vi "dust_event_query.vi"(6 "No. of Events":u64=10, 8 "error in (no error)":errorcluster, 9 "Limited?":bool, 10 "Small?":bool, 11 "Constraints":T4 {"Estimate Quality" scale=0.0..5.0; "Lower Mass Limit (kg)" min=-1.0 max=1.0 step=1e-20; "Upper Mass Limit (kg)" min=-1.0 max=1.0 step=1e-20; "Lower Velocity Limit (km/s)" min=-1.0 max=299792000.0; "Upper Velocity Limit (km/s)" min=-1.0 max=299792000.0}) -> (0 "error out":errorcluster, 1 "Experiment Settings ID Array":i32[](array[numeric]), 2 "Dust Event ID Array":i64[](array[numeric]), 3 "Dust Array":T1[](array[typedef]) {"File Location" items=["Unknown"=-1, "Processing"=0, "Storage"=1]; "Estimate Source" items=["Any Source."=-2, "No Shot"=-1, "Basic Labview Estimate"=0, "IDL Estimate From Andrew"=1, "IDL Estimate From Tobin"=2, "Old Metadata"=3]}, 5 "File Location Array":i8[](array[numeric]))   [LabVIEW 2013]
doc: "Given a set of constraints, this program will return a lot of data about each event that matches the constraints."
uses:
  User Interface/Controls/Constraints.ctl
  User Interface/Controls/Query_Dust_Event.ctl
  User Interface/Controls/Estimate_source.ctl
  User Interface/Controls/File_location.ctl
  <userlib>/_OpenG.lib/array/array.llb/Reverse 2D Array (Variant)__ogtk.vi
  <vilib>/addons/database/_DB Variant To Data/Database Variant To Data.xnode
panel:
  out "SQL Query Syntax":string
  # "Dust Event"
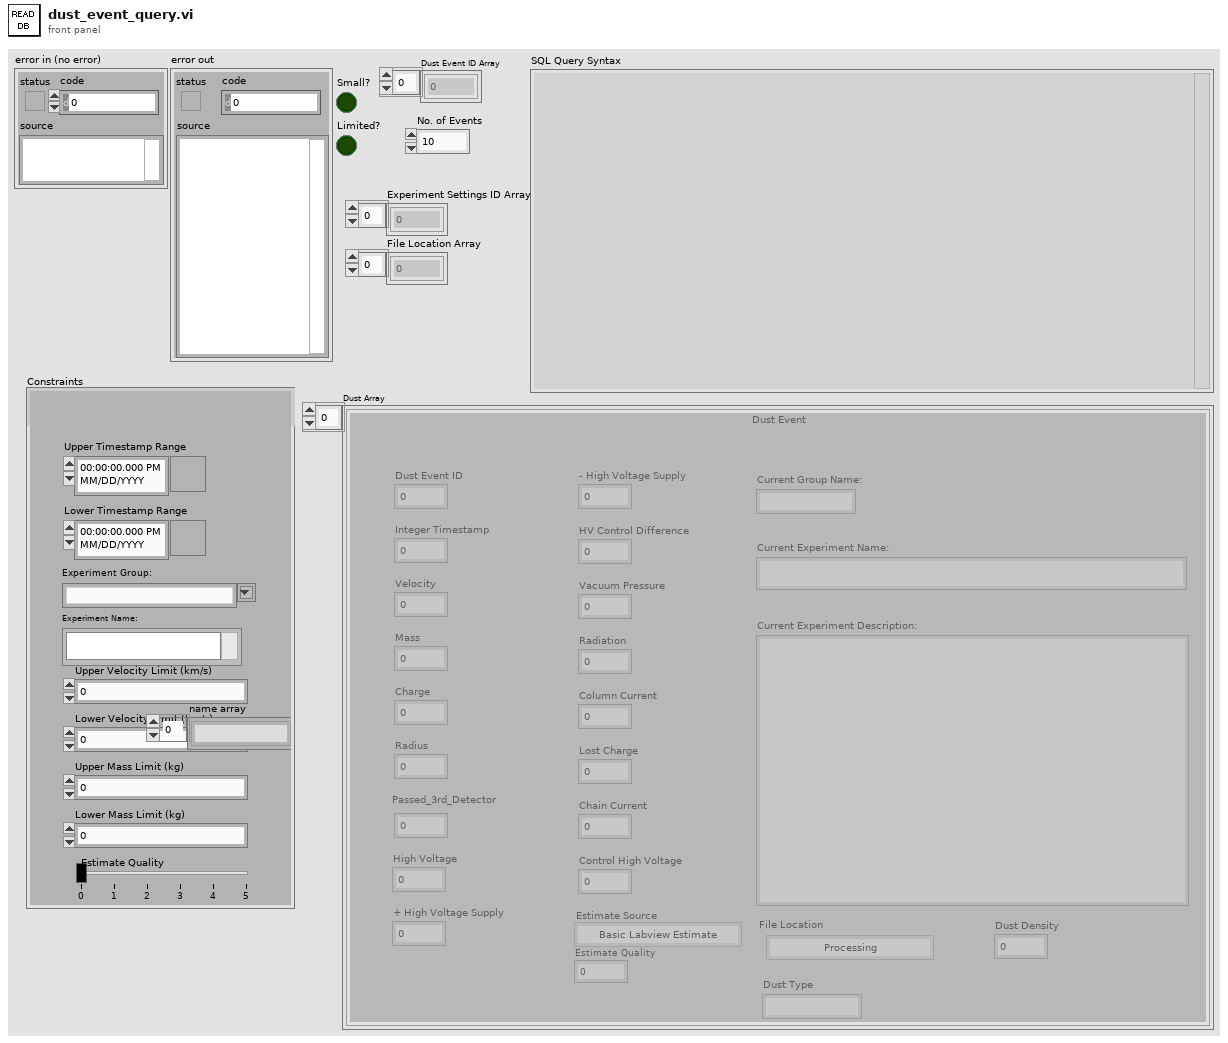
[diagram p1: front panel]
types:
  T1 = typedef "Query_Dust_Event.ctl" = cluster{"Dust Event ID":i64, "Integer Timestamp":i64, "Velocity":dbl, "Mass":dbl, "Charge":sgl, "Radius":sgl, "Passed_3rd_Detector":i8, "High Voltage":sgl, "+ High Voltage Supply":sgl, "- High Voltage Supply":sgl, "HV Control Difference":sgl, "Vacuum Pressure":sgl, "Radiation":sgl, "Column Current":sgl, "Lost Charge":sgl, "Chain Current":sgl, "Control High Voltage":sgl, "Current Group Name:":string, "Current Experiment Name:":string, "Current Experiment Description:":string, "Estimate Source":T2, "Estimate Quality":i8, "File Location":T3, "Dust Type":string, "Dust Density":sgl}
  T2 = typedef "Estimate_source.ctl" = i8
  T3 = typedef "File_location.ctl" = i8
  T4 = typedef "Constraints.ctl" = cluster{"Upper Timestamp Range":timestamp, "Lower Timestamp Range":timestamp, "Experiment Group:":string, "Experiment Name:":i32[], "Upper Velocity Limit (km/s)":dbl, "Lower Velocity Limit (km/s)":dbl, "Upper Mass Limit (kg)":dbl, "Lower Mass Limit (kg)":dbl, "name array":string[], "Estimate Quality":cluster{dbl, dbl}}
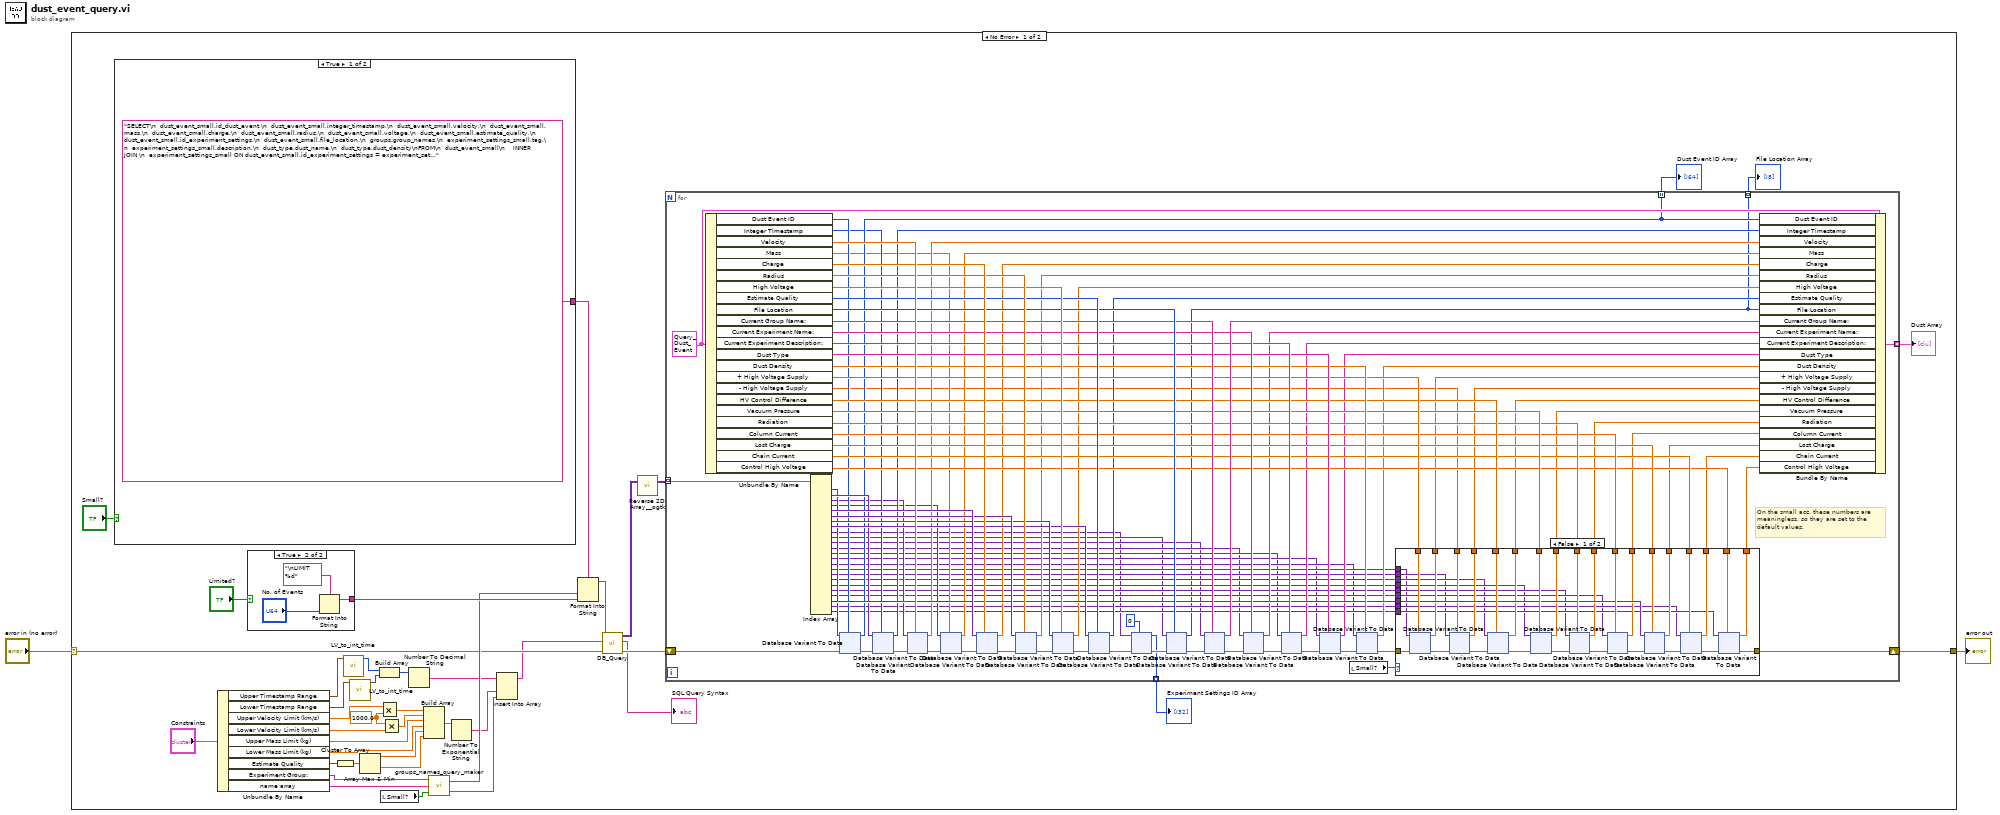
[diagram p0: block diagram]
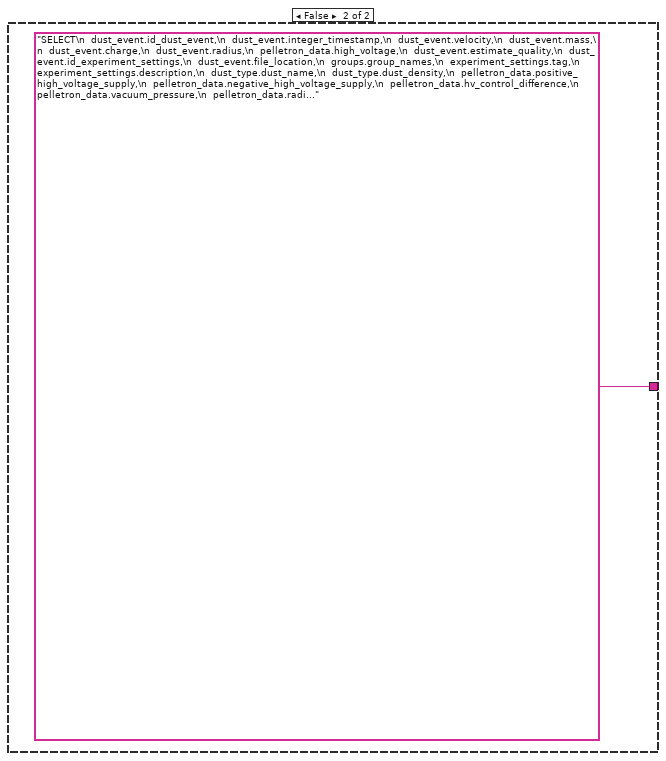
[diagram p3: hidden frame]
diagram:
  n1 = case shown="No Error" "error in (no error)" {
    selector: "error in (no error)" -> [w17 w957]
    tunnel: [w38 w957] -> w1
    frame No Error {
      w23 = 1000.0 ("y")
      n2 = case shown="True" "Small?" {
        tunnel: ["SELECT\n  dust_event_small.id_dust_event,\n  dust_event_small.integer_timestamp,\n  dust_event_small.velocity,\n  dust_event_small.mass,\n  dust_event_small.charge,\n  dust_event_small.radius,\n  dust_event_small.voltage,\n  dust_event_small.estimate_quality,\n  dust_event_small.id_experiment_settings,\n  dust_event_small.file_location,\n  groups.group_names,\n  experiment_settings_small.tag,\n  experiment_settings_small.description,\n  dust_type.dust_name,\n  dust_type.dust_density\nFROM\n  dust_event_small\n    INNER JOIN \n  experiment_settings_small ON dust_event_small.id_experiment_settings = experiment_settings_small.id_experiment_settings\n    INNER JOIN  \n  groups ON experiment_settings_small.id_groups=groups.id_groups\n    INNER JOIN\n  dust_info_small ON dust_event_small.id_dust_info = dust_info_small.id_dust_info\n  \t\tINNER JOIN\n  dust_type ON dust_info_small.dust_type = dust_type.id_dust_type\nWHERE\n  dust_event_small.integer_timestamp <= ? AND dust_event_small.integer_timestamp >= ?\n    AND\n  dust_event_small.velocity <= ? AND dust_event_small.velocity >= ?\n    AND\n  dust_event_small.mass <= ? AND dust_event_small.mass >= ?\n    AND\n  dust_event_small.estimate_quality <= ? AND dust_event_small.estimate_quality >= ?%s\nORDER BY\n  dust_event_small.id_dust_event DESC%s; " ("string") "SELECT\n  dust_event.id_dust_event,\n  dust_event.integer_timestamp,\n  dust_event.velocity,\n  dust_event.mass,\n  dust_event.charge,\n  dust_event.radius,\n  pelletron_data.high_voltage,\n  dust_event.estimate_quality,\n  dust_event.id_experiment_settings,\n  dust_event.file_location,\n  groups.group_names,\n  experiment_settings.tag,\n  experiment_settings.description,\n  dust_type.dust_name,\n  dust_type.dust_density,\n  pelletron_data.positive_high_voltage_supply,\n  pelletron_data.negative_high_voltage_supply,\n  pelletron_data.hv_control_difference,\n  pelletron_data.vacuum_pressure,\n  pelletron_data.radiation,\n  pelletron_data.column_current,\n  pelletron_data.lost_charge,\n  pelletron_data.chain_current,\n  pelletron_data.control_high_voltage\nFROM\n  dust_event\n    INNER JOIN \n  experiment_settings ON dust_event.id_experiment_settings = experiment_settings.id_experiment_settings\n    INNER JOIN  \n  groups ON experiment_settings.id_groups=groups.id_groups\n    INNER JOIN\n  pelletron_data ON pelletron_data.id_pelletron_data = dust_event.id_pelletron_data\n    INNER JOIN\n  dust_info ON dust_event.id_dust_info = dust_info.id_dust_info\n\t\t  INNER JOIN\n\t dust_type ON dust_info.dust_type = dust_type.id_dust_type\nWHERE\n  dust_event.integer_timestamp <= ?  AND dust_event.integer_timestamp >= ?\n    AND\n  dust_event.velocity <= ?  AND dust_event.velocity >= ?\n    AND\n  dust_event.mass <= ?  AND dust_event.mass >= ?\n    AND\n  dust_event.estimate_quality <= ? AND dust_event.estimate_quality >= ?%s\nORDER BY\n  dust_event.id_dust_event DESC%s; " ("string")] -> w29
        frame True {
        }
        frame False {
        }
      }
      n3 = Unbundle By Name("Constraints") -> ("Upper Timestamp Range"=w37:timestamp, "Lower Timestamp Range"=w36:timestamp, "Upper Velocity Limit (km/s)"=w35:dbl, "Lower Velocity Limit (km/s)"=w22:dbl, "Upper Mass Limit (kg)"=w11:dbl, "Lower Mass Limit (kg)"=w12:dbl, "Estimate Quality"=w24:cluster{dbl, dbl}, "Experiment Group:"=w26:string, "name array"=w25:string[])
      n4 = case shown="True" "Limited?" {
        tunnel: [_ w44] -> w28
        frame False {
        }
        frame True {
          n5 = Format Into String(format string="\nLIMIT %d", "No. of Events") -> (resulting string=w44:string)  [unwired: 2 in, 1 out]
        }
      }
      n6 = Cluster To Array(cluster=w24) -> (array=w40:dbl[])
      n7 = call "LV_to_int_time.vi"("Time Stamp"=w37) -> ("Integer Time"=w10:i64)  [unwired: 8 in, 1 out]
      n8 = call "LV_to_int_time.vi"("Time Stamp"=w36) -> ("Integer Time"=w9:i64)  [unwired: 8 in, 1 out]
      n9 = Array Max & Min(array=w40) -> (max value=w13:dbl, min value=w14:dbl)  [unwired: 2 out]
      n10 = Build Array(w10, w9) -> (w7:i64[])
      n11 = Multiply(x=w35, y=w23) -> (x*y=w16:dbl)
      n12 = local read "Small?"() -> (w18:bool)
      n13 = Multiply(x=w23, y=w22) -> (x*y=w15:dbl)
      n14 = Number To Decimal String(number=w7) -> (decimal integer string=w6:string[])  [unwired: 1 in]
      n15 = Build Array(w16, w15, w11, w12, w13, w14) -> (w8:dbl[])
      n16 = call "groups_names_query_maker.vi"("Small?"=w18, "Name Array"=w25, "Group  Name"=w26) -> ("Parameters"=w5:string[], "Group and Names Query"=w27:string)
      n17 = Number To Exponential String(number=w8) -> (E-format string=w4:string[])  [unwired: 3 in]
      n18 = Insert Into Array(array=w6, new element #1=w4, new element #2=w5) -> (w3:string[])  [unwired: 1 in]
      n19 = Format Into String(format string=w29, w27, w28) -> (resulting string=w21:string)  [unwired: 2 in, 1 out]
      n20 = call "DB_Query.vi"("error in (no error)"=w17, "Parameters"=w3, "Parameterized Query"=w21) -> ("error out"=w32:errorcluster, "Query in Standard Format"=→"SQL Query Syntax":string, "Results"=w31:variant[][])  [unwired: 6 in]
      n21 = call-poly <userlib>:"Reverse 2D Array__ogtk.vi"("Array"=w31) -> ("Reversed Array"=w33:variant[][])  [unwired: 2 in]
      n22 = for {
        tunnel: w33 -> [w141] mode=indexing
        shift-right: [w109] -> w38
        shift-left: w32 -> [w140]
        tunnel: [w114] -> w43 mode=indexing
        tunnel: [w101] -> w41 mode=indexing
        tunnel: [w51] -> w20 mode=indexing
        tunnel: [w50] -> w19 mode=indexing
        w139 = T1 {"Dust Event ID"=0, "Integer Timestamp"=0, "Velocity"=0.0, "Mass"=0.0, "Charge"=0.0, "Radius"=0.0, "Passed_3rd_Detector"=0, "High Voltage"=0.0, "+ High Voltage Supply"=0.0, "- High Voltage Supply"=0.0, "HV Control Difference"=0.0, "Vacuum Pressure"=0.0, "Radiation"=0.0, "Column Current"=0.0, "Lost Charge"=0.0, "Chain Current"=0.0, "Control High Voltage"=0.0, "Current Group Name:"="", "Current Experiment Name:"="", "Current Experiment Description:"="", "Estimate Source"=0, "Estimate Quality"=0, "File Location"=0, "Dust Type"="", "Dust Density"=0.0} ("Cluster")
        # "On the small acc, these numbers are\nmeaningless, so they are set to the\ndefault values."
        n23 = Unbundle By Name(w139) -> ("Dust Event ID"=w102:i64, "Integer Timestamp"=w100:i64, "Velocity"=w137:dbl, "Mass"=w95:dbl, "Charge"=w134:sgl, "Radius"=w130:sgl, "High Voltage"=w128:sgl, "Estimate Quality"=w126:i8, "File Location"=w125:T3, "Current Group Name:"=w124:string, "Current Experiment Name:"=w122:string, "Current Experiment Description:"=w121:string, "Dust Type"=w120:string, "Dust Density"=w119:sgl, "+ High Voltage Supply"=w118:sgl, "- High Voltage Supply"=w84:sgl, "HV Control Difference"=w117:sgl, "Vacuum Pressure"=w116:sgl, "Radiation"=w115:sgl, "Column Current"=w113:sgl, "Lost Charge"=w112:sgl, "Chain Current"=w111:sgl, "Control High Voltage"=w110:sgl)
        n24 = Index Array(array=w141) -> (element #1=w103:variant, element #2=w104:variant, element #3=w98:variant, element #4=w96:variant, element #5=w133:variant, element #6=w129:variant, element #7=w107:variant, element #8=w106:variant, element #9=w52:variant, element #10=w56:variant, element #11=w57:variant, element #12=w58:variant, element #13=w59:variant, element #14=w60:variant, element #15=w61:variant, element #16=w62:variant, element #17=w63:variant, element #18=w64:variant, element #19=w65:variant, element #20=w66:variant, element #21=w67:variant, element #22=w105:variant, element #23=w74:variant, element #24=w75:variant)  [unwired: 24 in]
        n25 = xnode "Database Variant To Data"("database variant"=w103, "error in (no error)"=w140, "type"=w102) -> ("data"=w101:i64, "error out"=w138:errorcluster)
        n26 = xnode "Database Variant To Data"("database variant"=w104, "error in (no error)"=w138, "type"=w100) -> ("data"=w99:i64, "error out"=w136:errorcluster)
        n27 = xnode "Database Variant To Data"("database variant"=w98, "error in (no error)"=w136, "type"=w137) -> ("data"=w97:dbl, "error out"=w135:errorcluster)
        n28 = xnode "Database Variant To Data"("database variant"=w96, "error in (no error)"=w135, "type"=w95) -> ("data"=w94:dbl, "error out"=w132:errorcluster)
        n29 = xnode "Database Variant To Data"("database variant"=w133, "error in (no error)"=w132, "type"=w134) -> ("data"=w93:sgl, "error out"=w131:errorcluster)
        n30 = xnode "Database Variant To Data"("database variant"=w129, "error in (no error)"=w131, "type"=w130) -> ("data"=w92:sgl, "error out"=w108:errorcluster)
        n31 = xnode "Database Variant To Data"("database variant"=w107, "error in (no error)"=w108, "type"=w128) -> ("data"=w91:sgl, "error out"=w127:errorcluster)
        n32 = xnode "Database Variant To Data"("database variant"=w106, "error in (no error)"=w127, "type"=w126) -> ("data"=w90:i8, "error out"=w54:errorcluster)
        n33 = xnode "Database Variant To Data"("database variant"=w52, "error in (no error)"=w54, "type"=0 ("data")) -> ("data"=w51:i32, "error out"=w55:errorcluster)
        n34 = xnode "Database Variant To Data"("database variant"=w56, "error in (no error)"=w55, "type"=w125) -> ("data"=w50:T3, "error out"=w73:errorcluster)
        n35 = xnode "Database Variant To Data"("database variant"=w57, "error in (no error)"=w73, "type"=w124) -> ("data"=w123:string, "error out"=w72:errorcluster)
        n36 = xnode "Database Variant To Data"("database variant"=w58, "error in (no error)"=w72, "type"=w122) -> ("data"=w89:string, "error out"=w71:errorcluster)
        n37 = xnode "Database Variant To Data"("database variant"=w59, "error in (no error)"=w71, "type"=w121) -> ("data"=w88:string, "error out"=w70:errorcluster)
        n38 = xnode "Database Variant To Data"("database variant"=w60, "error in (no error)"=w70, "type"=w120) -> ("data"=w87:string, "error out"=w69:errorcluster)
        n39 = local read "Small?"() -> (w49:bool)
        n40 = xnode "Database Variant To Data"("database variant"=w61, "error in (no error)"=w69, "type"=w119) -> ("data"=w86:sgl, "error out"=w68:errorcluster)
        n41 = case shown="False" w49 {
          tunnel: w118 -> [w178 w476]
          tunnel: w117 -> [w176 w474]
          tunnel: w116 -> [w174 w473]
          tunnel: w115 -> [w173 w472]
          tunnel: w113 -> [w172 w471]
          tunnel: w112 -> [w171 w470]
          tunnel: w111 -> [w169 w469]
          tunnel: w110 -> [w168 w468]
          tunnel: [w166 w467] -> w109
          tunnel: w105 -> [w163 _]
          tunnel: [w162 w476] -> w85
          tunnel: w84 -> [w161 w475]
          tunnel: [w160 w475] -> w83
          tunnel: [w159 w474] -> w82
          tunnel: [w158 w473] -> w81
          tunnel: [w157 w472] -> w80
          tunnel: [w156 w471] -> w79
          tunnel: [w155 w470] -> w78
          tunnel: [w154 w469] -> w77
          tunnel: [w153 w468] -> w76
          tunnel: w75 -> [w152 _]
          tunnel: w74 -> [w151 _]
          tunnel: w68 -> [w150 w467]
          tunnel: w67 -> [w147 _]
          tunnel: w66 -> [w146 _]
          tunnel: w65 -> [w145 _]
          tunnel: w64 -> [w144 _]
          tunnel: w63 -> [w143 _]
          tunnel: w62 -> [w142 _]
          frame False {
            n42 = xnode "Database Variant To Data"("database variant"=w142, "error in (no error)"=w150, "type"=w178) -> ("data"=w162:sgl, "error out"=w149:errorcluster)
            n43 = xnode "Database Variant To Data"("database variant"=w143, "error in (no error)"=w149, "type"=w161) -> ("data"=w160:sgl, "error out"=w177:errorcluster)
            n44 = xnode "Database Variant To Data"("database variant"=w144, "error in (no error)"=w177, "type"=w176) -> ("data"=w159:sgl, "error out"=w175:errorcluster)
            n45 = xnode "Database Variant To Data"("database variant"=w145, "error in (no error)"=w175, "type"=w174) -> ("data"=w158:sgl, "error out"=w164:errorcluster)
            n46 = xnode "Database Variant To Data"("database variant"=w146, "error in (no error)"=w164, "type"=w173) -> ("data"=w157:sgl, "error out"=w165:errorcluster)
            n47 = xnode "Database Variant To Data"("database variant"=w147, "error in (no error)"=w165, "type"=w172) -> ("data"=w156:sgl, "error out"=w148:errorcluster)
            n48 = xnode "Database Variant To Data"("database variant"=w163, "error in (no error)"=w148, "type"=w171) -> ("data"=w155:sgl, "error out"=w167:errorcluster)
            n49 = xnode "Database Variant To Data"("database variant"=w151, "error in (no error)"=w167, "type"=w169) -> ("data"=w154:sgl, "error out"=w170:errorcluster)
            n50 = xnode "Database Variant To Data"("database variant"=w152, "error in (no error)"=w170, "type"=w168) -> ("data"=w153:sgl, "error out"=w166:errorcluster)
          }
          frame True {
          }
        }
        n51 = Bundle By Name(cluster=w139, "Dust Event ID"=w101, "Integer Timestamp"=w99, "Velocity"=w97, "Mass"=w94, "Charge"=w93, "Radius"=w92, "High Voltage"=w91, "Estimate Quality"=w90, "File Location"=w50, "Current Group Name:"=w123, "Current Experiment Name:"=w89, "Current Experiment Description:"=w88, "Dust Type"=w87, "Dust Density"=w86, "+ High Voltage Supply"=w85, "- High Voltage Supply"=w83, "HV Control Difference"=w82, "Vacuum Pressure"=w81, "Radiation"=w80, "Column Current"=w79, "Lost Charge"=w78, "Chain Current"=w77, "Control High Voltage"=w76) -> (w114:T1)
      }
      "Dust Array" <- w43
      "Dust Event ID Array" <- w41
      "Experiment Settings ID Array" <- w20
      "File Location Array" <- w19
    }
    frame Error {
    }
  }
  "error out" <- w1
